vi "odczytajPrzyspieszenie.vi"(8 "Error In":errorcluster, 10 "I2C Adres":u8=24 format="%.0x", 11 "LINX Resource":T1={"IO"=enum."Remote", "Interface"=enum."TCP", "LINX Device Config"={"Interface"=enum."TCP", "COM Port"="N/A", "TCP Configuration"={"IP Address"="panicattack", "Port"=6999}, "Device Family"=4, "Device ID"=1, "Device Name"="Raspberry Pi Model B", "TCP Ref"=refnum, "Channels"={"DI"=[2, 3, 4, 7, 8, 9, 10, 11, 14, 15, 17, 18, 22, 23, 24, 25, 27], "DO"=[2, 3, 4, 7, 8, 9, 10, 11, 14, 15, 17, 18, 22, 23, 24, 25, 27], "AI"=[], "AO"=[], "PWM"=[], "QE"=[], "UART"=[0], "I2C 2"=[0, 1], "SPI"=[0], "CAN"=[], "Servo"=[], "AI Ref (V)"=0.0, "AI Resolution (Bits)"=0, "AO Ref (V)"=0.0, "AO Resolution (Bits)"=0}}}) -> (0 "Error Out":errorcluster, 2 "K¹ty nachylenia (st.)":dbl[](array[numeric]), 3 "LINX Resource 2":T1)   [LabVIEW 2014]
uses:
  <vilib>/MakerHub/LINX/Private/Type Defs/LINX Ref.ctl
  <vilib>/MakerHub/LINX/Private/Type Defs/Platform.ctl
  <vilib>/MakerHub/LINX/Private/Type Defs/Interface.ctl
  <vilib>/MakerHub/LINX/Private/Device/Type Defs/LINX Device Config.ctl
  <vilib>/MakerHub/LINX/Private/Device/Type Defs/TCP Config.ctl
  <vilib>/MakerHub/LINX/Private/Device/Type Defs/Channels.ctl
  <vilib>/MakerHub/LINX/Private/Local IO/LinxI2cWrite.vi
  <vilib>/MakerHub/LINX/Public/Utilities/Check Channel.vi
  <vilib>/MakerHub/LINX/Private/Utilties/Generate Error.vi
  <vilib>/MakerHub/LINX/LMH-LINX.lvlib
  <vilib>/MakerHub/LINX/Private/Device/Device.lvlib
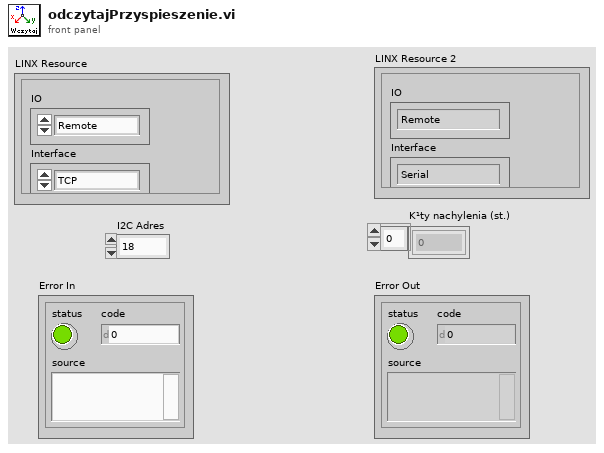
[diagram p1: front panel]
types:
  T1 = typedef "LMH-LINX.lvlib/LINX Ref.ctl" = cluster{"IO":T2, "Interface":T3, "LINX Device Config":T4}
  T2 = typedef "LMH-LINX.lvlib/Platform.ctl" = enum16{"Remote", "Local"}
  T3 = typedef "LMH-LINX.lvlib/Interface.ctl" = enum16{"Serial", "TCP"}
  T4 = typedef "LMH-LINX.lvlib/Device.lvlib/LINX Device Config.ctl" = cluster{"Interface":T3, "COM Port":refnum<visa-resource-name>, "TCP Configuration":T5, "Device Family":u8, "Device ID":u8, "Device Name":string, "TCP Ref":refnum<k5>, "Channels":T6}
  T5 = typedef "LMH-LINX.lvlib/Device.lvlib/TCP Config.ctl" = cluster{"IP Address":string, "Port":u16}
  T6 = typedef "LMH-LINX.lvlib/Channels.ctl" = cluster{"DI":u8[], "DO":u8[], "AI":u8[], "AO":u8[], "PWM":u8[], "QE":u8[], "UART":u8[], "I2C 2":u8[], "SPI":u8[], "CAN":u8[], "Servo":u8[], "AI Ref (V)":dbl, "AI Resolution (Bits)":u8, "AO Ref (V)":dbl, "AO Resolution (Bits)":u8}
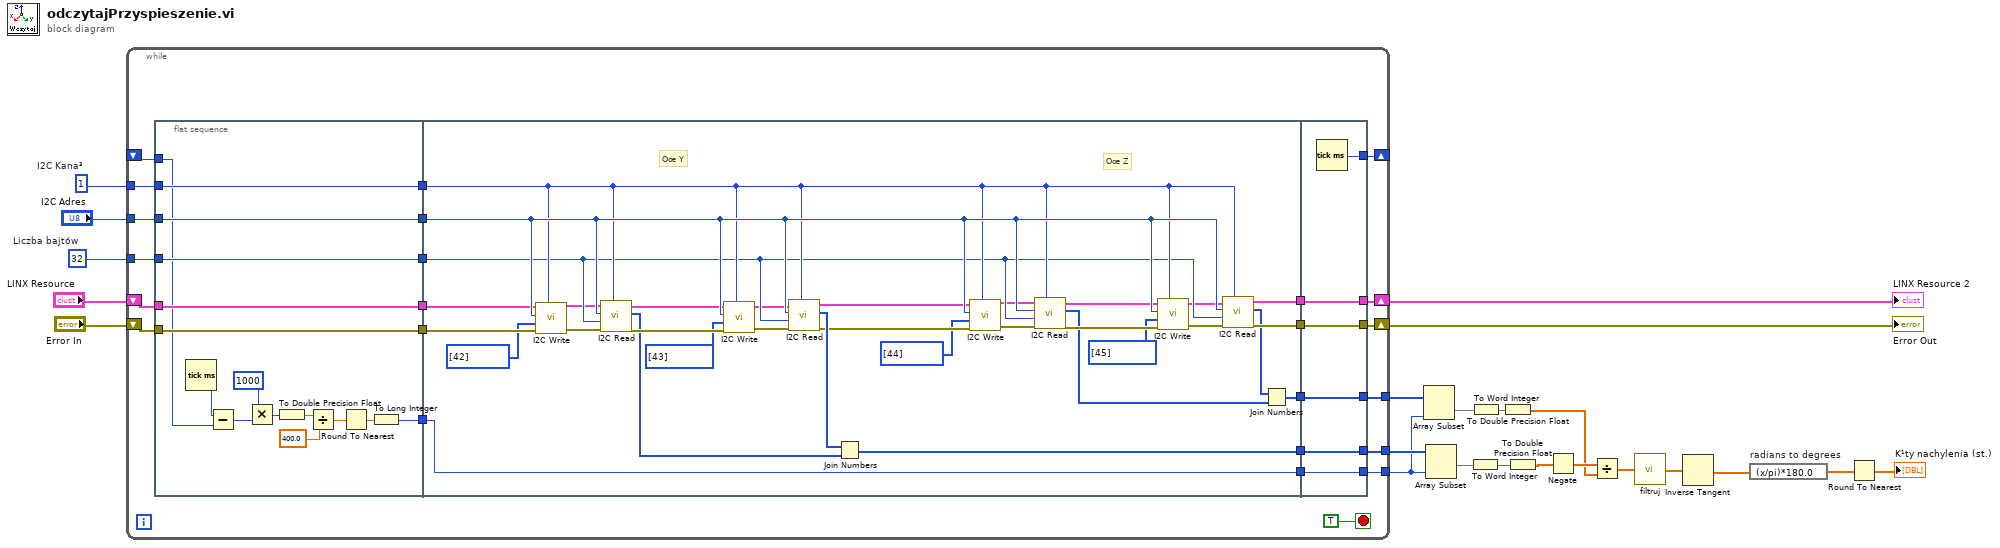
[diagram p0: block diagram]
diagram:
  w21 = u8 1  # I2C Kana³
  w20 = u8 32  # Liczba bajtów
  n1 = while {
    tunnel: "I2C Adres" -> [w46]
    tunnel: w21 -> [w45]
    tunnel: w20 -> [w44]
    tunnel: [w41] -> w17
    tunnel: [w38] -> w12
    shift-right: [w39] -> w15
    shift-left: "LINX Resource" -> [w43]
    shift-right: [w40] -> w16
    shift-left: "Error In" -> [w42]
    shift-right: [w33] -> _
    shift-left: _ -> [w26]
    tunnel: [w23] -> w3
    stop <- TRUE stop-if-true
    n2 = flat-sequence {
      tunnel: w42 -> [w57]
      tunnel: w43 -> [w58]
      tunnel: w44 -> [w59]
      tunnel: w45 -> [w60]
      tunnel: w46 -> [w61]
      tunnel: [w61] -> w31
      tunnel: [w60] -> w30
      tunnel: [w59] -> w29
      tunnel: [w58] -> w28
      tunnel: [w57] -> w27
      tunnel: w26 -> [w48]
      tunnel: [w47] -> w25
      tunnel: [w88] -> w37
      tunnel: [w87] -> w36
      tunnel: [w86] -> w35
      tunnel: [w85] -> w34
      tunnel: w31 -> [w93]
      tunnel: w30 -> [w92]
      tunnel: w29 -> [w91]
      tunnel: w28 -> [w90]
      tunnel: w27 -> [w89]
      tunnel: w25 -> [w62]
      tunnel: [w62] -> w24
      tunnel: [w96] -> w38
      tunnel: [w97] -> w39
      tunnel: [w98] -> w40
      tunnel: [w99] -> w41
      tunnel: w37 -> [w99]
      tunnel: w36 -> [w98]
      tunnel: w35 -> [w97]
      tunnel: w34 -> [w96]
      tunnel: [w95] -> w33
      tunnel: [w94] -> w23
      tunnel: w24 -> [w94]
      frame #0 {
        n3 = Tick Count (ms)() -> (millisecond timer value=w49:u32)
        n4 = Subtract(x=w49, y=w48) -> (x-y=w50:u32)
        n5 = Multiply(x=u32 1000, y=w50) -> (x*y=w54:u32)
        n6 = To Double Precision Float(number=w54) -> (double precision float=w55:dbl)
        n7 = Divide(x=w55, y=400.0) -> (x/y=w53:dbl)
        n8 = Round To Nearest(number=w53) -> (nearest integer value=w56:dbl)
        n9 = To Long Integer(number=w56) -> (32bit integer=w47:i32)
      }
      frame #1 {
        # "Oœ Z"
        # "Oœ Y"
        n10 = call <vilib>:"I2C Write.vi"("I2C Channel"=w92, "Error In"=w89, "Data"=u8[] [42], "I2C Slave Address (0)"=w93, "LINX Resource"=w90) -> ("Error Out"=w82:errorcluster, "LINX Resource"=w83:T1)  [unwired: 5 in]
        n11 = call <vilib>:"I2C Read.vi"("I2C Channel"=w92, "Error In"=w82, "Bytes To Read"=w91, "I2C Slave Address (0)"=w93, "LINX Resource"=w83) -> ("Error Out"=w79:errorcluster, "Data"=w76:u8[], "LINX Resource"=w80:T1)  [unwired: 4 in]
        n12 = call <vilib>:"I2C Write.vi"("I2C Channel"=w92, "Error In"=w79, "Data"=u8[] [43], "I2C Slave Address (0)"=w93, "LINX Resource"=w80) -> ("Error Out"=w81:errorcluster, "LINX Resource"=w78:T1)  [unwired: 5 in]
        n13 = call <vilib>:"I2C Read.vi"("I2C Channel"=w92, "Error In"=w81, "Bytes To Read"=w91, "I2C Slave Address (0)"=w93, "LINX Resource"=w78) -> ("Error Out"=w68:errorcluster, "Data"=w77:u8[], "LINX Resource"=w69:T1)  [unwired: 4 in]
        n14 = Join Numbers(hi=w77, lo=w76) -> ((hi.lo)=w85:u16[])
        n15 = call <vilib>:"I2C Write.vi"("I2C Channel"=w92, "Error In"=w68, "Data"=u8[] [44], "I2C Slave Address (0)"=w93, "LINX Resource"=w69) -> ("Error Out"=w74:errorcluster, "LINX Resource"=w75:T1)  [unwired: 5 in]
        n16 = call <vilib>:"I2C Read.vi"("I2C Channel"=w92, "Error In"=w74, "Bytes To Read"=w91, "I2C Slave Address (0)"=w93, "LINX Resource"=w75) -> ("Error Out"=w71:errorcluster, "Data"=w66:u8[], "LINX Resource"=w72:T1)  [unwired: 4 in]
        n17 = call <vilib>:"I2C Write.vi"("I2C Channel"=w92, "Error In"=w71, "Data"=u8[] [45], "I2C Slave Address (0)"=w93, "LINX Resource"=w72) -> ("Error Out"=w73:errorcluster, "LINX Resource"=w70:T1)  [unwired: 5 in]
        n18 = call <vilib>:"I2C Read.vi"("I2C Channel"=w92, "Error In"=w73, "Bytes To Read"=w91, "I2C Slave Address (0)"=w93, "LINX Resource"=w70) -> ("Error Out"=w87:errorcluster, "Data"=w67:u8[], "LINX Resource"=w86:T1)  [unwired: 4 in]
        n19 = Join Numbers(hi=w67, lo=w66) -> ((hi.lo)=w88:u16[])
      }
      frame #2 {
        n20 = Tick Count (ms)() -> (millisecond timer value=w95:u32)
      }
    }
  }
  "Error Out" <- w16
  "LINX Resource 2" <- w15
  n21 = Array Subset(array=w17, length=w3) -> (w6:u16[])  [unwired: 1 in]
  n22 = Array Subset(array=w12, length=w3) -> (w10:u16[])  [unwired: 1 in]
  n23 = To Word Integer(number=w10) -> (16bit integer=w9:i16[])
  n24 = To Word Integer(number=w6) -> (16bit integer=w7:i16[])
  n25 = To Double Precision Float(number=w7) -> (double precision float=w5:dbl[])
  n26 = To Double Precision Float(number=w9) -> (double precision float=w8:dbl[])
  n27 = Negate(x=w8) -> (-x=w11:dbl[])
  n28 = Divide(x=w11, y=w5) -> (x/y=w2:dbl[])
  n29 = call "filtruj.vi"("tab. wejœciowa"=w2) -> ("tab. przefiltrowana"=w1:dbl[])  [unwired: 4 in]
  n30 = Inverse Tangent(1:w1) -> (0:w13:dbl[])
  n31 = expression code="(x/pi)*180.0" "radians to degrees"(w13) -> (w14:dbl[])
  n32 = Round To Nearest(number=w14) -> (nearest integer value=→"K¹ty nachylenia (st.)":dbl[])
